vi "TEST_RemoteCmds.vi"   [LabVIEW 2012]
panel:
  # "Open the diagram to see the code executing\n\nLED 1 should blink 10 times\n\nPush PB3 to rerun program, PB1 to abort it, and PB5 to see your IP address"
types:
  T1 = typedef "URAPI_Control.ctl" = cluster{"Script":string, "Whiles":u8[], "Ifs":u8[], "Supress Err":bool, "Errors":string}
  T2 = typedef "BotSpeak_Control.ctl" = cluster{"Address":string, "Reply EOF":string, "Hardware":path, "Retries":i8, "Timeout":i32}
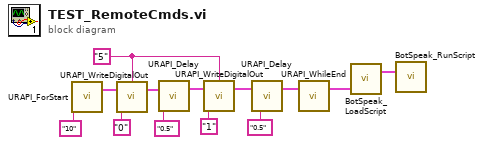
[diagram p0: block diagram]
diagram:
  w3 = "5" ("Channel")
  n1 = call <userlib>:"URAPI_ForStart.vi"("Iterations"="10") -> ("URAPI Script Out"=w13:T1)  [unwired: 3 in, 1 out]
  n2 = call <userlib>:"URAPI_WriteDigitalOut.vi"("Variable In"="0", "URAPI Script"=w13, "Channel"=w3) -> ("URAPI Script"=w11:T1)  [unwired: 1 in, 1 out]
  n3 = call <userlib>:"URAPI_Delay.vi"("Variable In"="0.5", "URAPI Script"=w11) -> ("URAPI Script out"=w9:T1)  [unwired: 3 in]
  n4 = call <userlib>:"URAPI_WriteDigitalOut.vi"("Variable In"="1", "URAPI Script"=w9, "Channel"=w3) -> ("URAPI Script"=w8:T1)  [unwired: 1 in, 1 out]
  n5 = call <userlib>:"URAPI_Delay.vi"("Variable In"="0.5", "URAPI Script"=w8) -> ("URAPI Script out"=w5:T1)  [unwired: 3 in]
  n6 = call <userlib>:"URAPI_WhileEnd.vi"("URAPI Script"=w5) -> ("URAPI Script Out"=w2:T1)  [unwired: 4 in]
  n7 = call <userlib>:"BotSpeak_LoadScript.vi"("URAPI Script"=w2) -> ("Bot Settings"=w1:T2)  [unwired: 1 in, 1 out]
  n8 = call <userlib>:"BotSpeak_RunScript.vi"("Bot Settings"=w1) -> ()  [unwired: 1 in, 2 out]
